vi "Launch Object by Type Response.vi"(5 "Enqueuer":refnum<class "Message Enqueuer.lvclass">, 6 "Requestor":string, 8 "error in (no error)":errorcluster, 9 "Name":string, 10 "Type":string, 11 "Da Base in":refnum<class "Da Base.lvclass">) -> (0 "error out":errorcluster, 3 "Da Base out":refnum<class "Da Base.lvclass">)   [LabVIEW 2016, in "Da Base.lvclass"]
uses:
  Da Base.lvclass
  <vilib>/ActorFramework/Message Enqueuer/Message Enqueuer.lvclass
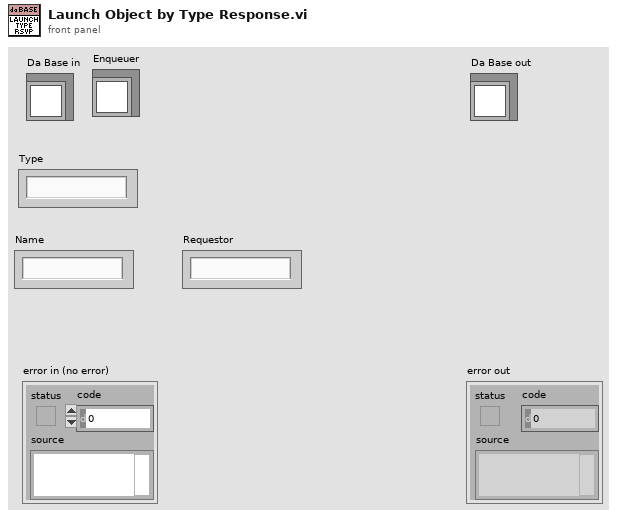
[diagram p1: front panel]
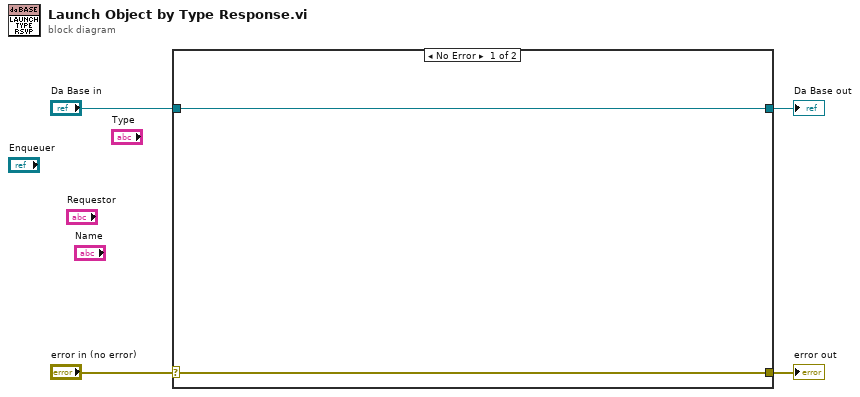
[diagram p0: block diagram]
diagram:
  n1 = case shown="No Error" "error in (no error)" {
    selector: "error in (no error)" -> [w5 w8]
    tunnel: [w5 w8] -> w3
    tunnel: [w6 w7] -> w1
    tunnel: "Da Base in" -> [w6 w7]
    frame No Error {
    }
    frame Error {
    }
  }
  "error out" <- w3
  "Da Base out" <- w1
